vi "Inicio_BIn.vi"(0 "Refnum in":refnum<k21>, 5 "error in (no error)":errorcluster) -> (14 "Refnum out":refnum<k21>, 19 "error out":errorcluster)   [LabVIEW 2013]
uses:
  <vilib>/DAQmx/write.llb/DAQmx Write (Digital U32 1Chan 1Samp).vi
  <vilib>/DAQmx/miscellaneous.llb/DAQmx Fill In Error Info.vi
panel:
  out "number":u32
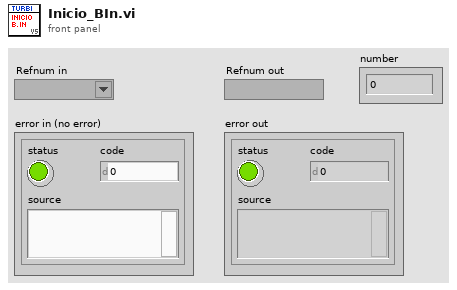
[diagram p1: front panel]
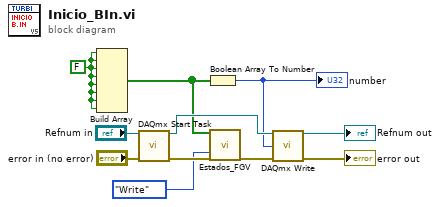
[diagram p0: block diagram]
diagram:
  w5 = FALSE
  n1 = Build Array(w5, w5, w5, w5, w5, w5, w5, w5) -> (w1:bool[])
  n2 = call <vilib>:"DAQmx Start Task.vi"("task/channels in"="Refnum in", "error in"="error in (no error)") -> ("task out"=w9:refnum<k21>, "error out"=w4:errorcluster)  [unwired: 12 in]
  n3 = Boolean Array To Number(Boolean array=w1) -> (number=w6:u32)
  "number" <- w6
  n4 = call "Estados_FGV.vi"("Estados_IN"=w1, "Opción"=enum16{"Write", "Read"}."Write", "Error In"=w4) -> ("Error Out"=w3:errorcluster)  [unwired: 15 in, 1 out]
  n5 = call-poly <vilib>:"DAQmx Write.vi"("task/channels in"=w9, "data"=w6, "error in"=w3) -> ("task out"=→"Refnum out":refnum<k21>, "error out"=→"error out":errorcluster)  [unwired: 10 in, 1 out]
